vi "Real_Average.vi"(6 "new input spectrum":dbl[](array[numeric]), 8 "old input array":dbl[][](array[numeric]), 10 "Number of averages":i32, 11 "current measurement number":i32) -> (0 "output array":dbl[][](array[numeric]), 3 "next measurement number":i32, 4 "output spectrum":dbl[](array[numeric]))   [LabVIEW 2013]
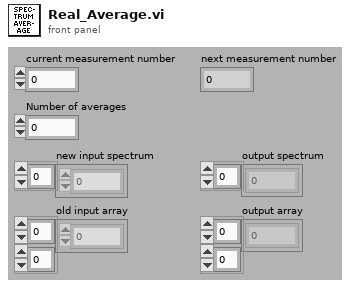
[diagram p1: front panel]
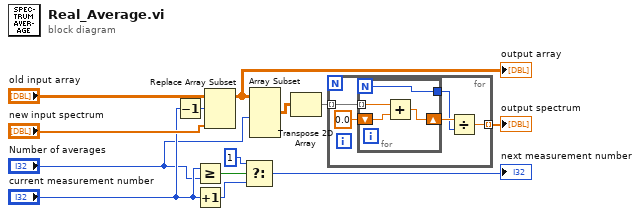
[diagram p0: block diagram]
diagram:
  n1 = Decrement(x="current measurement number") -> (x-1=w6:i32)
  n2 = Greater Or Equal?(x="current measurement number", y="Number of averages") -> (x >= y?=w11:bool)
  n3 = Increment(x="current measurement number") -> (x+1=w12:i32)
  n4 = Replace Array Subset(array="old input array", new element="new input spectrum", index (row)=w6) -> (w3:dbl[][])  [unwired: 1 in]
  "output array" <- w3
  n5 = Select(t=1, s=w11, f=w12) -> (s? t:f=→"next measurement number":i32)
  n6 = Array Subset(array=w3, length (row)="Number of averages") -> (w2:dbl[][])  [unwired: 3 in]
  n7 = Transpose 2D Array(2D array=w2) -> (transposed array=w5:dbl[][])
  n8 = for {
    tunnel: w5 -> [w14] mode=indexing
    tunnel: [w15] -> w4 mode=indexing
    n9 = for {
      N -> [w20]
      tunnel: w14 -> [w19] mode=indexing
      shift-right: [w21] -> w17
      shift-left: 0.0 -> [w22]
      tunnel: [w20] -> w16
      n10 = Add(x=w19, y=w22) -> (x+y=w21:dbl)
    }
    n11 = Divide(x=w17, y=w16) -> (x/y=w15:dbl)
  }
  "output spectrum" <- w4
